vi "TestExec.Configure Reports, Lookup Rpt Dir.vi"(10 "Seq Name":string, 11 "Seq_Dir":cluster{"Sequence":string, "Folder":path}[](array[cluster])) -> (3 "Folder":path)   [LabVIEW 2018]
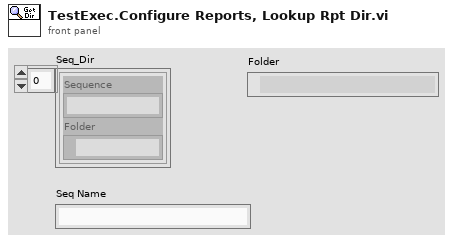
[diagram p1: front panel]
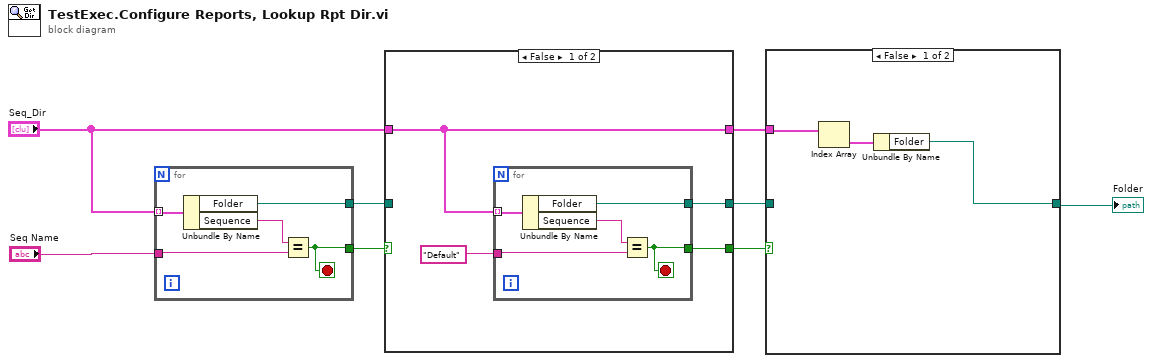
[diagram p0: block diagram]
diagram:
  n1 = for {
    tunnel: "Seq_Dir" -> [w13] mode=indexing
    tunnel: "Seq Name" -> [w11]
    tunnel: [w10] -> w6
    tunnel: [w9] -> w5
    stop <- w10 stop-if-true
    n2 = Unbundle By Name(w13) -> ("Folder"=w9:path, "Sequence"=w12:string)
    n3 = Equal?(x=w12, y=w11) -> (x = y?=w10:bool)
  }
  n4 = case shown="False" w6 {
    selector: w6 -> [_ w24]
    tunnel: "Seq_Dir" -> [w14 w23]
    tunnel: w5 -> [_ w25]
    tunnel: [w16 w25] -> w3
    tunnel: [w15 w24] -> w4
    tunnel: [w14 w23] -> w2
    frame False {
      n5 = for {
        tunnel: w14 -> [w22] mode=indexing
        tunnel: "Default" -> [w20]
        tunnel: [w19] -> w15
        tunnel: [w18] -> w16
        stop <- w19 stop-if-true
        n6 = Unbundle By Name(w22) -> ("Folder"=w18:path, "Sequence"=w21:string)
        n7 = Equal?(x=w21, y=w20) -> (x = y?=w19:bool)
      }
    }
    frame True {
    }
  }
  n8 = case shown="False" w4 {
    tunnel: w3 -> [_ w29]
    tunnel: [w26 w29] -> w1
    tunnel: w2 -> [w28 _]
    frame False {
      n9 = Index Array(array=w28) -> (element=w27:cluster{"Sequence":string, "Folder":path})  [unwired: 1 in]
      n10 = Unbundle By Name(w27) -> ("Folder"=w26:path)
    }
    frame True {
    }
  }
  "Folder" <- w1
